vi "Convert State Enum to String.vi"(9 "state in":T1, 12 "error in":errorcluster) -> (10 "state out":string, 14 "error out":errorcluster)   [LabVIEW 2026, in "Synchronize AWS S3 Content.lvlib" / "Synchronize AWS S3 Content TLB`.lvclass"]
doc: "Convert State.ctl enum to a string.\n\n<B>Input Parameters</B>\n\n<B>state in</B> is the current state of the system of type enum.\n\n<B>error in</B> describes error conditions that occur before this node runs. This input provides standard error in functionality.\n\n<B>Output Parameters</B>\n\n<B>state out/B> is the current state of the system of type string.\n\n<B>error out</B> contains error information. This output provides standard error out functionality."
uses:
  Synchronize AWS S3 Content TLB`.lvclass
  State Machine/State.ctl
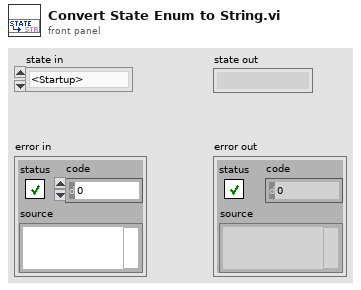
[diagram p1: front panel]
types:
  T1 = typedef "Synchronize AWS S3 Content.lvlib/Synchronize AWS S3 Content TLB`.lvclass/State.ctl" = enum16{"<Startup>", "Idle", "Initiating Configuration", "Validating Commands", "Executing Synchronization", "Validation", "<Shutdown>", "<Error>"}
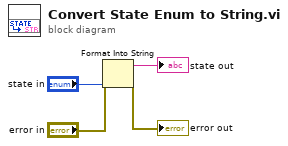
[diagram p0: block diagram]
diagram:
  n1 = Format Into String(error in="error in", "state in") -> (resulting string=→"state out":string, error out=→"error out":errorcluster)  [unwired: 2 in]
